vi "PyLoN_data2.vi"(7 "Number of Images":u32=1 min=1 step=1, 8 "error in (no error)":errorcluster, 9 "PumpOffBkgd":dbl[](array[numeric]), 10 "PumpOnBkgd":dbl[](array[numeric]), 11 "Camera Handle":u32) -> (0 "error out":errorcluster, 1 "Pump_Off":dbl[](array[numeric]), 2 "Pump_On":dbl[](array[numeric]), 3 "Camera Handle 2":u32 caption="Camera Handle", 4 "Raman_Gain":dbl[](array[numeric]), 5 "x/y":dbl)   [LabVIEW 2014]
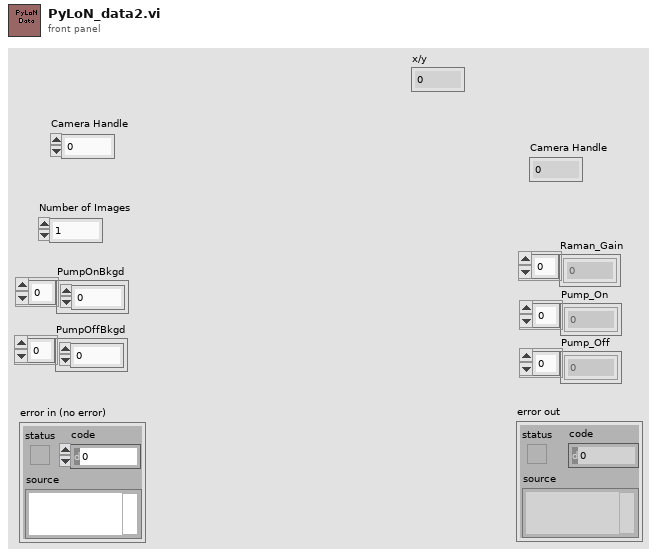
[diagram p1: front panel]
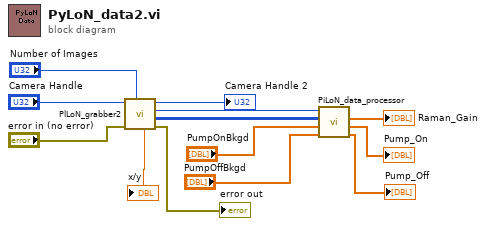
[diagram p0: block diagram]
diagram:
  n1 = call "PlLoN_grabber2.vi"("Number of Images"="Number of Images", "error in (no error)"="error in (no error)", "Camera Handle"="Camera Handle") -> ("error out"=→"error out":errorcluster, "DATA"=w12:u16[][], "Number of Images"=w13:u32, "Camera Handle"=→"Camera Handle 2":u32, "x/y"=→"x/y":dbl)  [unwired: 4 in]
  n2 = call "PiLoN_data_processor.vi"("PumpOffBkgd"="PumpOffBkgd", "PumpOnBkgd"="PumpOnBkgd", "Data"=w12, "# of Images"=w13) -> ("Pump_Off"=→"Pump_Off":dbl[], "Pump_On"=→"Pump_On":dbl[], "Raman_Gain"=→"Raman_Gain":dbl[])  [unwired: 5 in]
